vi "Get Scene Object Refnum.vi"(8 "error in (no error)":errorcluster, 11 "XRay Part Sample in":refnum<class "XRay Part Sample.lvclass">) -> (0 "error out":errorcluster, 2 "Part":refnum<vi>, 3 "XRay Part Sample out":refnum<class "XRay Part Sample.lvclass">)   [LabVIEW 2026, in "XRay Part Sample.lvclass"]
uses:
  XRay Part Sample.lvclass
  XRay Part Sample.lvclass/XRay Part Sample.ctl
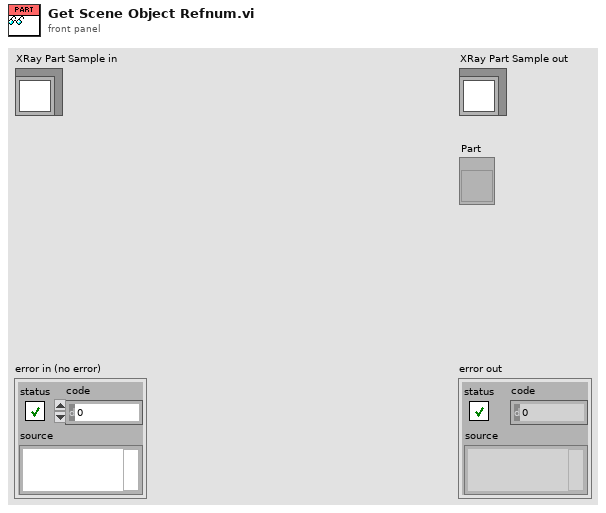
[diagram p1: front panel]
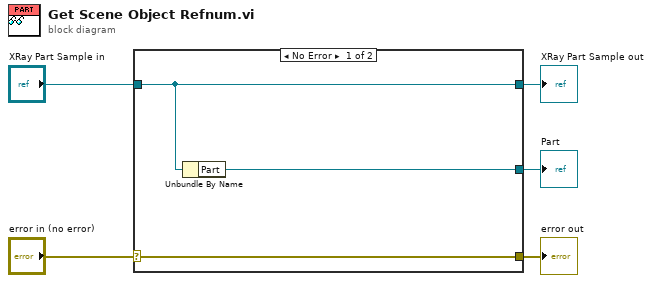
[diagram p0: block diagram]
diagram:
  n1 = case shown="No Error" "error in (no error)" {
    selector: "error in (no error)" -> [w8 w9]
    tunnel: [w8 w9] -> w4
    tunnel: [w7 w10] -> w2
    tunnel: "XRay Part Sample in" -> [w7 w10]
    tunnel: [w6 _] -> w1
    frame No Error {
      n2 = Unbundle By Name(w7) -> ("Part"=w6:refnum<vi>)
    }
    frame Error {
    }
  }
  "error out" <- w4
  "XRay Part Sample out" <- w2
  "Part" <- w1
